vi "speedDisplay.vi"(0 "refnum in":refnum<file>, 5 "VISA resource name":refnum<visa-resource-name>="COM11", 7 "MAX":string="10.0", 9 "E-Stop":bool, 11 "error in":errorcluster) -> (3 "FREQUENCY":string, 4 "SPEED":dbl(knob) scale=0.0..12.0, 6 "START":string, 8 "result":bool, 10 "MID":string, 14 "PWM":string, 15 "error out":errorcluster)   [LabVIEW 2018]
panel:
  out "MPH/KPH":string
  in  "lower limit":string="04.9"
  in  "upper limit":string="05.1"
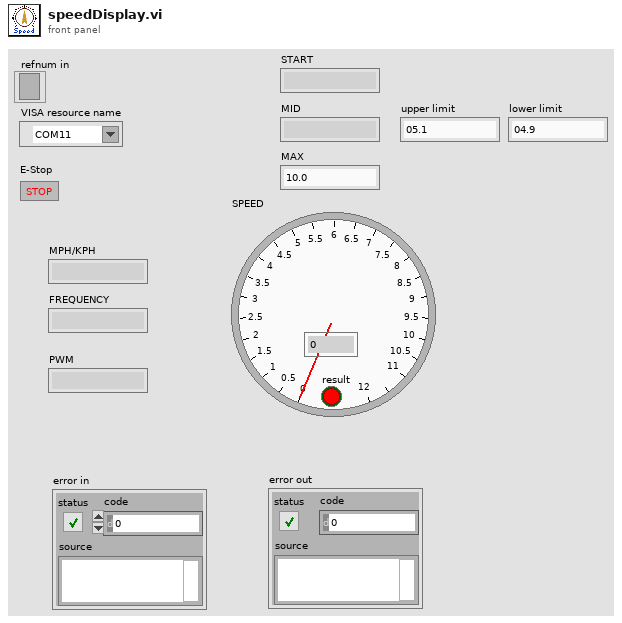
[diagram p1: front panel]
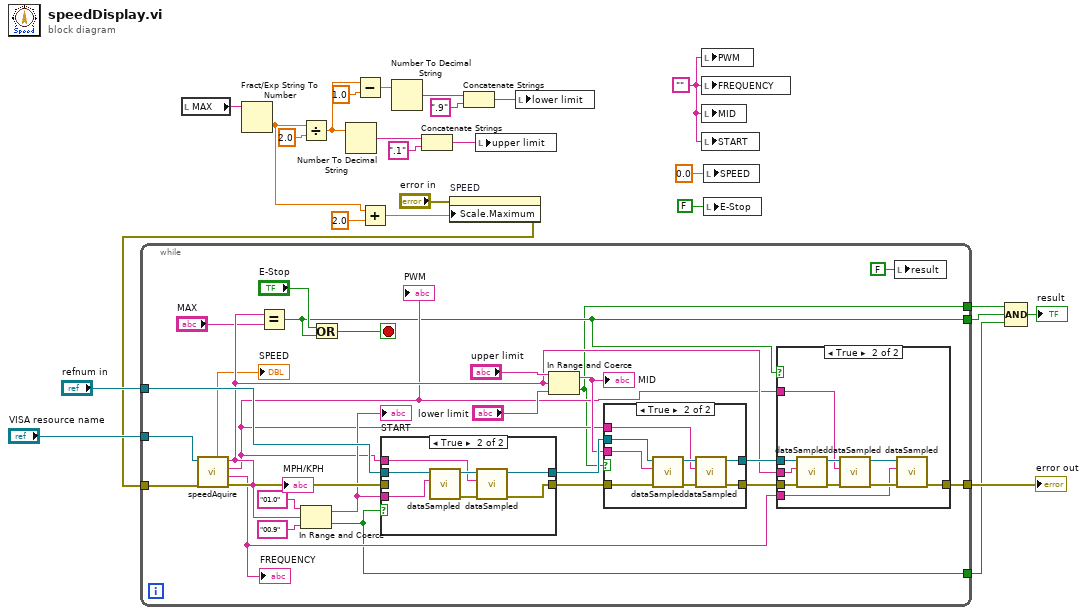
[diagram p0: block diagram]
diagram:
  w10 = ""
  n1 = local read "MAX"() -> (w21:string)
  n2 = Fract/Exp String To Number(string=w21) -> (number=w6:dbl)  [unwired: 3 in, 1 out]
  n3 = Divide(x=w6, y=2.0) -> (x/y=w14:dbl)
  n4 = Number To Decimal String(number=w14) -> (decimal integer string=w17:string)  [unwired: 1 in]
  n5 = Subtract(x=w14, y=1.0) -> (x-y=w15:dbl)
  n6 = Add(x=w6, y=2.0) -> (x+y=w5:dbl)
  n7 = Number To Decimal String(number=w15) -> (decimal integer string=w12:string)  [unwired: 1 in]
  n8 = Concatenate Strings(w17, ".1" ("string")) -> (w19:string)
  n9 = property on="SPEED" class="Knob (strict)"(error in="error in", "Scale.Maximum"=w5) -> (error out=w8:errorcluster)  [unwired: 1 in, 1 out]
  n10 = while {
    tunnel: "refnum in" -> [w44]
    tunnel: [w36] -> w23
    tunnel: "VISA resource name" -> [w35]
    tunnel: w8 -> [w33]
    tunnel: [w31] -> w2
    tunnel: [w30] -> w3
    tunnel: [w29] -> w4
    stop <- w42 stop-if-true
    n11 = call "speedAquire.vi"("error in (no error)"=w33, "VISA resource name"=w35) -> ("error out (no error)"=w43:errorcluster, "FREQUENCY"=w32:string, "PWM"=w34:string, "MPH/KPH"=w41:string, "SPEED"=→"SPEED":dbl)  [unwired: 5 in]
    "FREQUENCY" <- w32
    "PWM" <- w34
    "MPH/KPH" <- w41
    n12 = Equal?(x=w41, y="MAX") -> (x = y?=w30:bool)
    n13 = In Range and Coerce(upper limit="01.0", x=w41, lower limit="00.9") -> (coerced(x)=w38:string, In Range?=w31:bool)
    "START" <- w38
    n14 = Or(x="E-Stop", y=w30) -> (x .or. y?=w42:bool)
    n15 = case shown="True" w31 {
      tunnel: [w74 w76] -> w48
      tunnel: [w75 w78] -> w46
      tunnel: w44 -> [w75 w82]
      tunnel: w43 -> [w74 _]
      tunnel: w38 -> [_ w81]
      tunnel: w34 -> [_ w77]
      frame False {
      }
      frame True {
        n16 = call "dataSampled.vi"("Data"=w81, "refnum in"=w82) -> ("error out"=w80:errorcluster, "refnum out"=w79:refnum<file>)  [unwired: 8 in]
        n17 = call "dataSampled.vi"("Error In"=w80, "Data"=w77, "refnum in"=w79) -> ("error out"=w76:errorcluster, "refnum out"=w78:refnum<file>)  [unwired: 7 in]
      }
    }
    n18 = In Range and Coerce(upper limit="upper limit", x=w41, lower limit="lower limit") -> (coerced(x)=w39:string, In Range?=w29:bool)
    "MID" <- w39
    n19 = case shown="True" w29 {
      tunnel: [w64 w67] -> w47
      tunnel: w48 -> [w64 w73]
      tunnel: w46 -> [w65 w72]
      tunnel: [w65 w68] -> w45
      tunnel: w39 -> [_ w71]
      tunnel: w34 -> [_ w66]
      frame False {
      }
      frame True {
        n20 = call "dataSampled.vi"("Error In"=w73, "Data"=w71, "refnum in"=w72) -> ("error out"=w70:errorcluster, "refnum out"=w69:refnum<file>)  [unwired: 7 in]
        n21 = call "dataSampled.vi"("Error In"=w70, "Data"=w66, "refnum in"=w69) -> ("error out"=w67:errorcluster, "refnum out"=w68:refnum<file>)  [unwired: 7 in]
      }
    }
    n22 = case shown="True" w30 {
      tunnel: w47 -> [w53 w63]
      tunnel: w45 -> [_ w62]
      tunnel: w41 -> [_ w61]
      tunnel: [w53 w55] -> w36
      tunnel: w34 -> [_ w58]
      tunnel: w32 -> [_ w54]
      frame False {
      }
      frame True {
        n23 = call "dataSampled.vi"("Error In"=w63, "Data"=w61, "refnum in"=w62) -> ("error out"=w60:errorcluster, "refnum out"=w59:refnum<file>)  [unwired: 7 in]
        n24 = call "dataSampled.vi"("Error In"=w60, "Data"=w58, "refnum in"=w59) -> ("error out"=w57:errorcluster, "refnum out"=w56:refnum<file>)  [unwired: 7 in]
        n25 = call "dataSampled.vi"("Error In"=w57, "Data"=w54, "refnum in"=w56) -> ("error out"=w55:errorcluster)  [unwired: 7 in, 1 out]
      }
    }
    n26 = local write "result"(FALSE ("result")) -> ()
  }
  "error out" <- w23
  n27 = Concatenate Strings(w12, ".9" ("string")) -> (w18:string)
  n28 = local write "upper limit"(w19) -> ()
  n29 = local write "lower limit"(w18) -> ()
  n30 = local write "PWM"(w10) -> ()
  n31 = local write "FREQUENCY"(w10) -> ()
  n32 = local write "MID"(w10) -> ()
  n33 = local write "START"(w10) -> ()
  n34 = local write "SPEED"(0.0 ("SPEED")) -> ()
  n35 = local write "E-Stop"(FALSE ("stop")) -> ()
  n36 = Compound Arithmetic op=AND(w4, w3, w2) -> (→"result":bool)
